vi "FPGA_1.vi"() -> ()   [LabVIEW 2022 SP3]
uses:
  <vilib>/rvi/Emulation/niFpgaGetClockAttributes.vi
  <vilib>/rvi/Emulation/niFpgaSctlEmulationGetInTimedLoop.vi
  <vilib>/rvi/Emulation/niFpgaEmulationReportErrorSimple.vi
  <vilib>/rvi/eio/common/nirviEmuTemplateMethod_errors.vi
  <vilib>/rvi/Emulation/niFpgaCriticalErrorInLSC.vi
  <vilib>/eio/EIONode/EIONode.xnode
panel:
  in  "Mod1/DO13":bool
  in  "Mod1/DO12":bool
  in  "Mod1/DO11":bool
  in  "Mod1/DO10":bool
  in  "PWM_DO6":u32 caption="PWM DO6"
  in  "PWM_DO7":u32 caption="PWM DO7"
  in  "PWM_DO4":u32 caption="PWM DO4"
  in  "PWM_DO5":u32 caption="PWM DO5"
  in  "PWM_DO2":u32 caption="PWM DO2"
  in  "PWM_DO3":u32 caption="PWM DO3"
  in  "PWM_DO0":u32 caption="PWM DO0"
  out "Mod1/DI8":bool
  out "Mod1/DI7":bool
  out "Mod1/DI6":bool
  out "Mod1/DI5":bool
  out "Mod1/DI4":bool
  out "Mod1/DI3":bool
  out "Mod1/DI2":bool
  out "Mod1/DI1":bool
  out "Mod1/DI0":bool
  in  "PWM_DO1":u32 caption="PWM DO1"
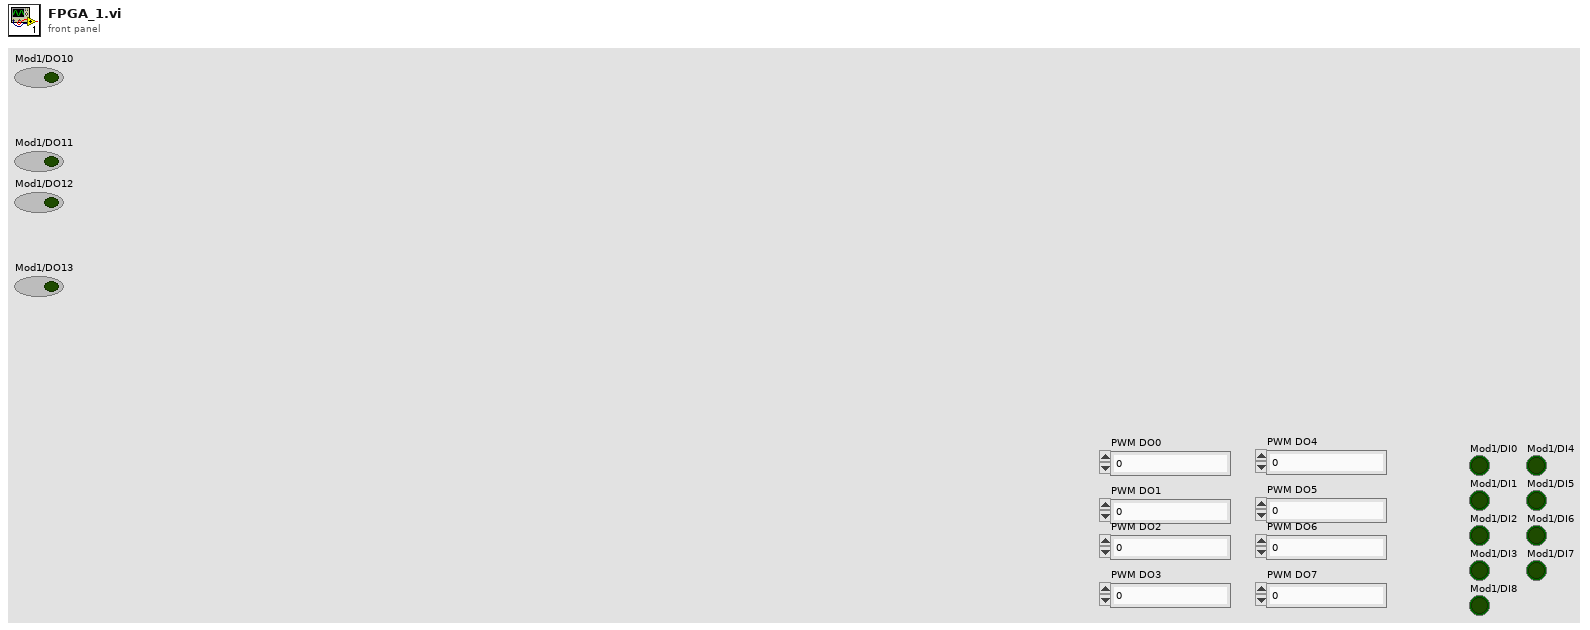
[diagram p1: front panel]
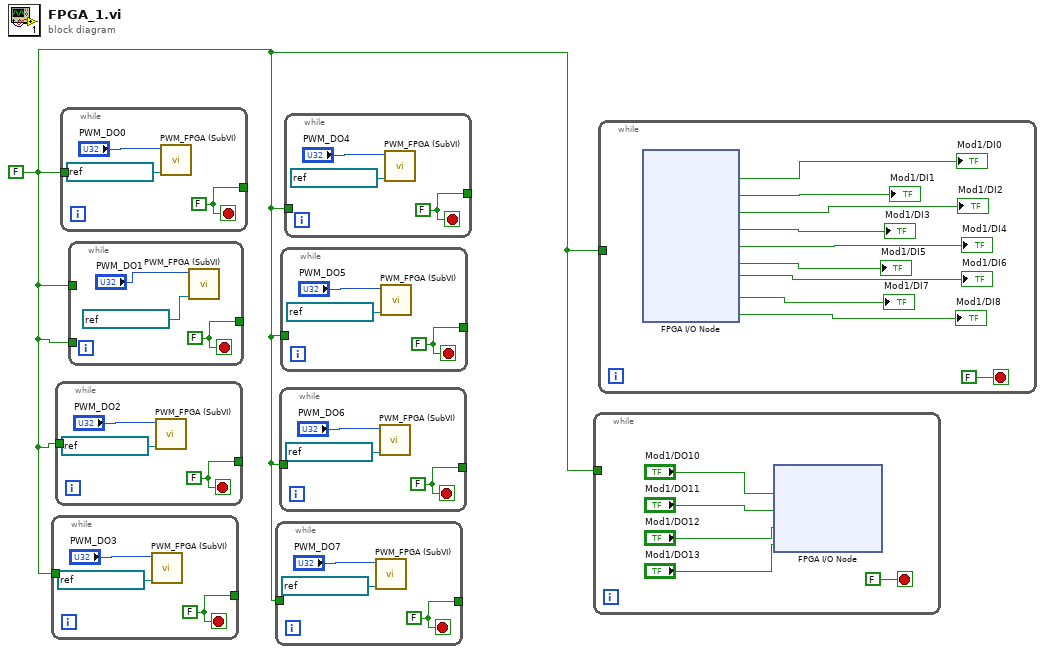
[diagram p0: block diagram]
diagram:
  w1 = FALSE
  n1 = while {
    tunnel: [w3] -> _
    tunnel: w1 -> [_]
    stop <- w3 stop-if-true
    w3 = FALSE
    n2 = call "PWM_FPGA (SubVI).vi"("FPGA I/O In"=refnum<k21> "Mod1/DO3", "PWM_IN_gen"="PWM_DO3") -> ()  [unwired: 10 in]
  }
  n3 = while {
    tunnel: [w6] -> _
    tunnel: w1 -> [_]
    stop <- w6 stop-if-true
    w6 = FALSE
    n4 = call "PWM_FPGA (SubVI).vi"("FPGA I/O In"=refnum<k21> "Mod1/DO2", "PWM_IN_gen"="PWM_DO2") -> ()  [unwired: 10 in]
  }
  n5 = while {
    tunnel: [w9] -> _
    tunnel: w1 -> [_]
    stop <- w9 stop-if-true
    w9 = FALSE
    n6 = call "PWM_FPGA (SubVI).vi"("FPGA I/O In"=refnum<k21> "Mod1/DO0", "PWM_IN_gen"="PWM_DO0") -> ()  [unwired: 10 in]
  }
  n7 = while {
    tunnel: [w12] -> _
    tunnel: w1 -> [_]
    tunnel: w1 -> [_]
    stop <- w12 stop-if-true
    w12 = FALSE
    n8 = call "PWM_FPGA (SubVI).vi"("FPGA I/O In"=refnum<k21> "Mod1/DO9", "PWM_IN_gen"="PWM_DO1") -> ()  [unwired: 10 in]
  }
  n9 = while {
    tunnel: [w15] -> _
    tunnel: w1 -> [_]
    stop <- w15 stop-if-true
    w15 = FALSE
    n10 = call "PWM_FPGA (SubVI).vi"("FPGA I/O In"=refnum<k21> "Mod1/DO7", "PWM_IN_gen"="PWM_DO7") -> ()  [unwired: 10 in]
  }
  n11 = while {
    tunnel: [w18] -> _
    tunnel: w1 -> [_]
    stop <- w18 stop-if-true
    w18 = FALSE
    n12 = call "PWM_FPGA (SubVI).vi"("FPGA I/O In"=refnum<k21> "Mod1/DO6", "PWM_IN_gen"="PWM_DO6") -> ()  [unwired: 10 in]
  }
  n13 = while {
    tunnel: [w21] -> _
    tunnel: w1 -> [_]
    stop <- w21 stop-if-true
    w21 = FALSE
    n14 = call "PWM_FPGA (SubVI).vi"("FPGA I/O In"=refnum<k21> "Mod1/DO5", "PWM_IN_gen"="PWM_DO5") -> ()  [unwired: 10 in]
  }
  n15 = while {
    tunnel: [w24] -> _
    tunnel: w1 -> [_]
    stop <- w24 stop-if-true
    w24 = FALSE
    n16 = call "PWM_FPGA (SubVI).vi"("FPGA I/O In"=refnum<k21> "Mod1/DO4", "PWM_IN_gen"="PWM_DO4") -> ()  [unwired: 10 in]
  }
  n17 = while {
    tunnel: w1 -> [_]
    stop <- FALSE stop-if-true
    n18 = xnode "FPGA I/O Node"("Mod1/DO10"="Mod1/DO10", "Mod1/DO11"="Mod1/DO11", "Mod1/DO12"="Mod1/DO12", "Mod1/DO13"="Mod1/DO13") -> ()  [unwired: 4 in, 4 out]
  }
  n19 = while {
    tunnel: w1 -> [_]
    stop <- FALSE stop-if-true
    n20 = xnode "FPGA I/O Node"() -> ("Mod1/DI0"=→"Mod1/DI0":bool, "Mod1/DI1"=→"Mod1/DI1":bool, "Mod1/DI2"=→"Mod1/DI2":bool, "Mod1/DI3"=→"Mod1/DI3":bool, "Mod1/DI4"=→"Mod1/DI4":bool, "Mod1/DI5"=→"Mod1/DI5":bool, "Mod1/DI6"=→"Mod1/DI6":bool, "Mod1/DI7"=→"Mod1/DI7":bool, "Mod1/DI8"=→"Mod1/DI8":bool)  [unwired: 9 in, 9 out]
  }
